vi "MSScript_Exe_Cmd_LoopCounting.vi"(7 "Function":enum16{"Init", "LoopStart", "LoopEnd"}(ring)=enum."LoopStart", 9 "Index":i32, 11 "Times":i32) -> (0 "Error?":bool, 1 "Index of the next sentence":i32)   [LabVIEW 2018, in "MSScript.lvclass"]
uses:
  MSScript.lvclass
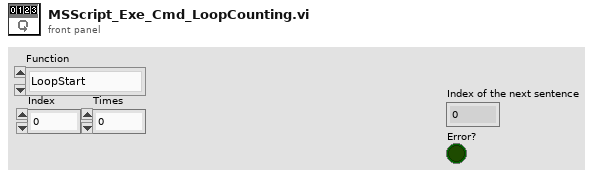
[diagram p1: front panel]
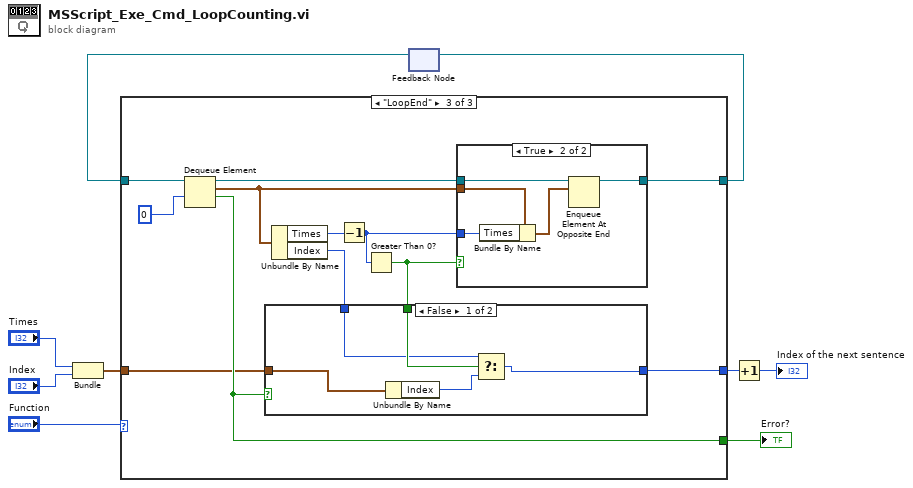
[diagram p0: block diagram]
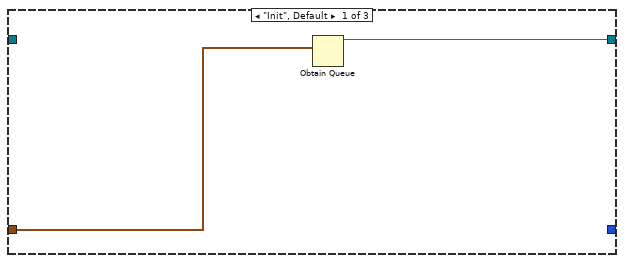
[diagram p2: hidden frame]
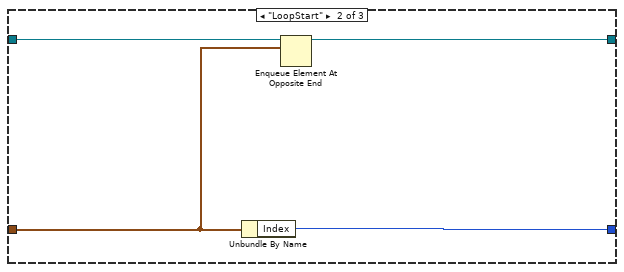
[diagram p3: hidden frame]
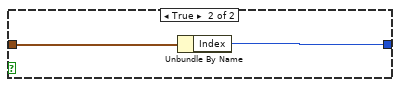
[diagram p4: hidden frame]
diagram:
  n1 = Bundle("Times"="Times", "Index"="Index") -> (w7:cluster{"Times":i32, "Index":i32})  [unwired: 1 in]
  n2 = feedback #1() -> (w5:refnum<queue>)  [unwired: 1 in]
  n3 = case shown="\"LoopEnd\"" "Function" {
    tunnel: w7 -> [w11 w13 w19]
    tunnel: [w10 w14 w23] -> w6
    tunnel: w5 -> [_ w15 w27]
    tunnel: [_ w12 w21] -> w3
    tunnel: [_ _ w20] -> w2
    frame "Init", Default {
      n4 = Obtain Queue(element data type=w11) -> (queue out=w10:refnum<queue>)  [unwired: 4 in, 2 out]
    }
    frame "LoopStart" {
      n5 = Unbundle By Name(w13) -> ("Index"=w12:i32)
      n6 = Enqueue Element At Opposite End(queue=w15, element=w13) -> (queue out=w14:refnum<queue>)  [unwired: 2 in, 2 out]
    }
    frame "LoopEnd" {
      n7 = Dequeue Element(queue=w27, timeout in ms (-1)=0) -> (queue out=w24:refnum<queue>, element=w25:cluster{"Times":i32, "Index":i32}, timed out?=w20:bool)  [unwired: 1 in, 1 out]
      n8 = Unbundle By Name(w25) -> ("Times"=w18:i32, "Index"=w22:i32)
      n9 = Decrement(x=w18) -> (x-1=w16:i32)
      n10 = Greater Than 0?(x=w16) -> (x > 0?=w17:bool)
      n11 = case shown="False" w20 {
        tunnel: w22 -> [w29 _]
        tunnel: [w28 w33] -> w21
        tunnel: w19 -> [w31 w34]
        tunnel: w17 -> [w32 _]
        frame False {
          n12 = Unbundle By Name(w31) -> ("Index"=w30:i32)
          n13 = Select(t=w29, s=w32, f=w30) -> (s? t:f=w28:i32)
        }
        frame True {
          n14 = Unbundle By Name(w34) -> ("Index"=w33:i32)
        }
      }
      n15 = case shown="True" w17 {
        tunnel: w25 -> [_ w40]
        tunnel: w16 -> [_ w39]
        tunnel: w24 -> [w35 w38]
        tunnel: [w35 w36] -> w23
        frame False {
        }
        frame True {
          n16 = Bundle By Name(cluster=w40, "Times"=w39) -> (w37:cluster{"Times":i32, "Index":i32})
          n17 = Enqueue Element At Opposite End(queue=w38, element=w37) -> (queue out=w36:refnum<queue>)  [unwired: 2 in, 2 out]
        }
      }
    }
  }
  "Error?" <- w2
  n18 = feedback-in #1(w6) -> ()
  n19 = Increment(x=w3) -> (x+1=→"Index of the next sentence":i32)
